vi "SupplyCHConfig.vi"(8 "error in (no error)":errorcluster caption="错误输入（无错误）", 9 "Voltage(V)":dbl=5.0, 10 "CH":enum16{"Positive", "Negative"}(ring), 11 "handle":u64) -> (0 "error out":errorcluster caption="错误输出", 2 "function return":i32, 3 "handle out":u64)   [LabVIEW 2018]
doc: "Set pos. or neg. Supply voltage"
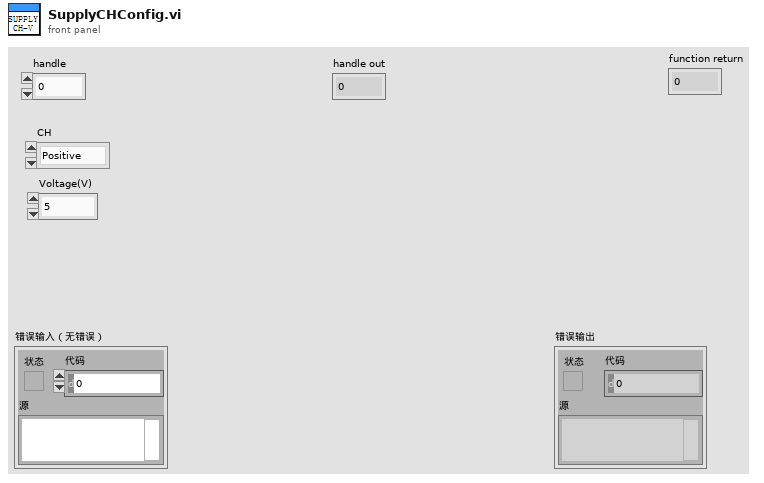
[diagram p1: front panel]
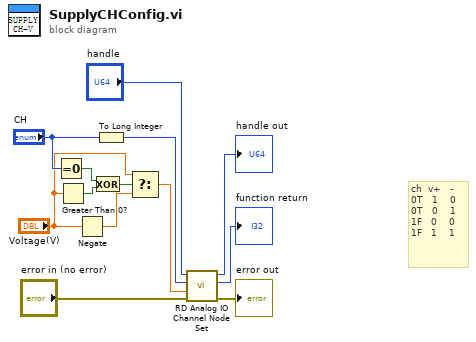
[diagram p0: block diagram]
diagram:
  # "ch  v+   -\n0T   1    0\n0T   0    1\n1F   0    0\n1F   1    1"
  n1 = Equal To 0?(x="CH") -> (x = 0?=w6:bool)
  n2 = Greater Than 0?(x="Voltage(V)") -> (x > 0?=w7:bool)
  n3 = Negate(x="Voltage(V)") -> (-x=w2:dbl)
  n4 = Exclusive Or(1:w7, 2:w6) -> (0:w5:bool)
  n5 = To Long Integer(number="CH") -> (32bit integer=w1:i32)
  n6 = Select(t="Voltage(V)", s=w5, f=w2) -> (s? t:f=w4:dbl)
  n7 = call "RD Analog IO Channel Node Set.vi"("error in (no error)"="error in (no error)", "value"=w4, "ch"=w1, "handle"="handle") -> ("error out"=→"error out":errorcluster, "function return"=→"function return":i32, "handle out"=→"handle out":u64)  [unwired: 4 in, 1 out]
